vi "display queue.vi"(7 "Action":T1=enum."Enqueue", 8 "error in (no error)":errorcluster, 10 "time out":i32=100, 11 "Array in":sgl[](array[numeric])) -> (0 "error out":errorcluster, 1 "Array out":sgl[](array[numeric]), 2 "Empty?":bool, 3 "timed out?":bool)   [LabVIEW 2018]
uses:
  Controls/Queue Manager Actions.ctl
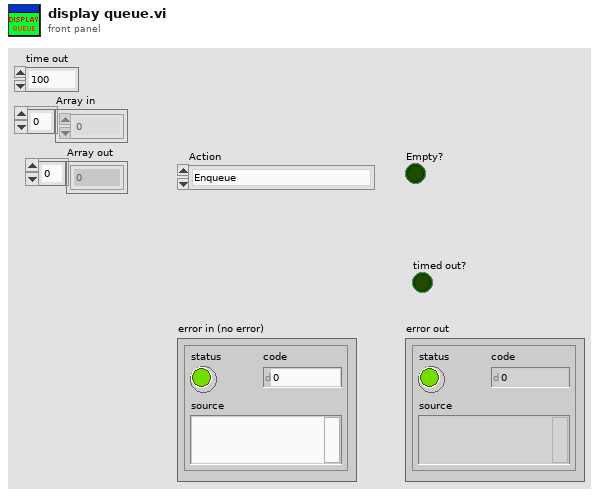
[diagram p1: front panel]
types:
  T1 = typedef "Queue Manager Actions.ctl" = enum16{"Init", "Enqueue", "Enqueue All", "Preview Queue", "Dequeue", "Get Status", "Flush Queue", "Flush All Queues", "Release All Queues", "Release Queue", "Enqueue at Opposite End"}
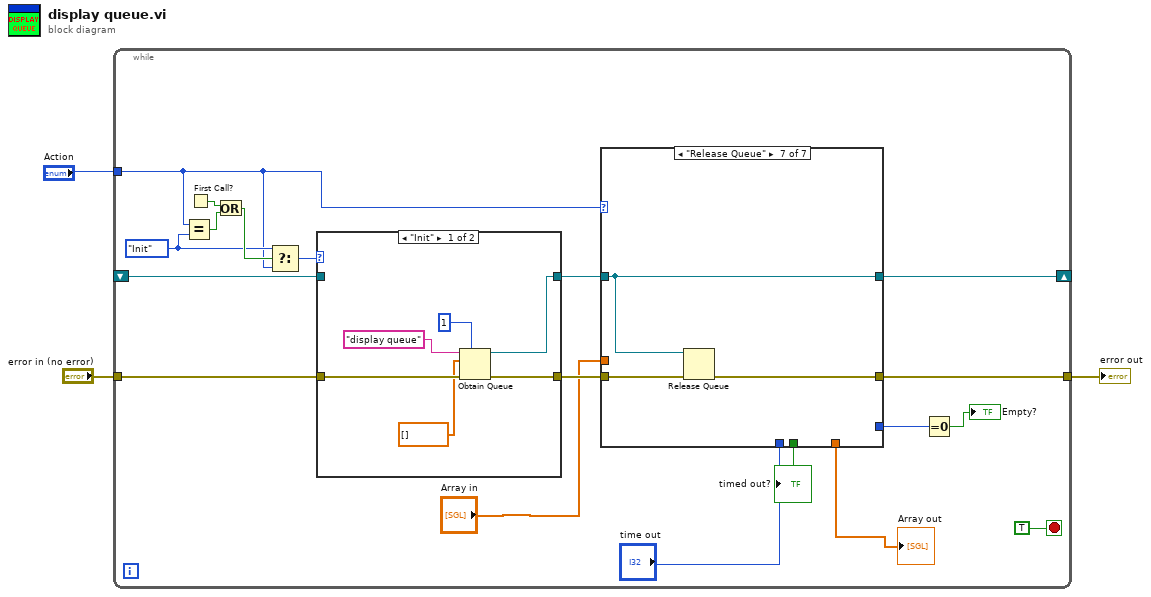
[diagram p0: block diagram]
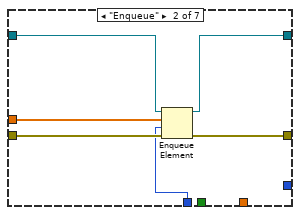
[diagram p3: hidden frame]
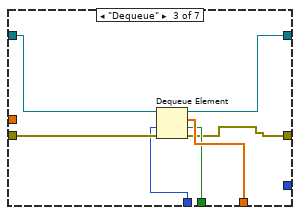
[diagram p4: hidden frame]
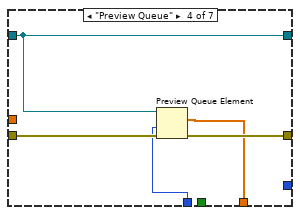
[diagram p5: hidden frame]
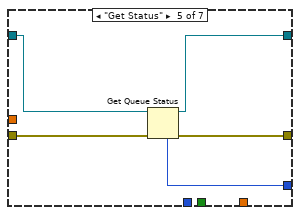
[diagram p6: hidden frame]
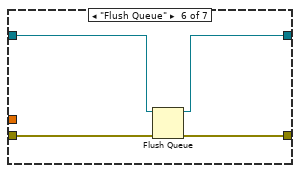
[diagram p7: hidden frame]
diagram:
  n1 = while {
    tunnel: "Action" -> [w10]
    tunnel: "error in (no error)" -> [w17]
    tunnel: [w16] -> w1
    shift-right: [w12] -> _
    shift-left: _ -> [w11]
    stop <- TRUE stop-if-true
    w19 = Queue_Manager_Actions."Init"
    n2 = Equal?(x=w10, y=w19) -> (x = y?=w21:bool)
    n3 = First Call?() -> (First Call?: T/F=w22:bool)
    n4 = Or(x=w22, y=w21) -> (x .or. y?=w20:bool)
    n5 = Select(t=w19, s=w20, f=w10) -> (s? t:f=w18:T1)
    n6 = case shown="\"Init\"" w18 {
      tunnel: [w60 w61] -> w14
      tunnel: w17 -> [w59 w62]
      tunnel: [w58 w62] -> w15
      tunnel: w11 -> [_ w61]
      frame "Init" {
        n7 = Obtain Queue(max queue size (-1, unlimited)=1, name (unnamed)="display queue" ("queue name"), element data type=sgl[] [], error in (no error)=w59) -> (queue out=w60:refnum<queue>, error out=w58:errorcluster)  [unwired: 1 in, 1 out]
      }
      frame "Enqueue", Default {
      }
    }
    n8 = case shown="\"Release Queue\"" w10 {
      tunnel: w14 -> [w23 w26 w35 w39 w45 w49 w52]
      tunnel: [w24 w29 w31 w41 w46 w50 w53] -> w16
      tunnel: w15 -> [w24 w30 w37 w42 w47 w51 w54]
      tunnel: [w23 w25 w32 w39 w44 w48 w52] -> w12
      tunnel: "time out" -> [_ w28 w36 w40 _ _ _]
      tunnel: "Array in" -> [_ w27 _ _ _ _ _]
      tunnel: [_ _ _ _ w43 _ _] -> w8
      tunnel: [_ _ w34 w38 _ _ _] -> w4
      tunnel: [_ _ w33 _ _ _ _] -> w7
      frame "Init", Default {
      }
      frame "Enqueue" {
        n9 = Enqueue Element(queue=w26, element=w27, timeout in ms (-1)=w28, error in (no error)=w30) -> (queue out=w25:refnum<queue>, error out=w29:errorcluster)  [unwired: 1 out]
      }
      frame "Dequeue" {
        n10 = Dequeue Element(queue=w35, timeout in ms (-1)=w36, error in (no error)=w37) -> (queue out=w32:refnum<queue>, element=w34:sgl[], timed out?=w33:bool, error out=w31:errorcluster)
      }
      frame "Preview Queue" {
        n11 = Preview Queue Element(queue=w39, timeout in ms (-1)=w40, error in (no error)=w42) -> (element=w38:sgl[], error out=w41:errorcluster)  [unwired: 2 out]
      }
      frame "Get Status" {
        n12 = Get Queue Status(queue=w45, error in (no error)=w47) -> (queue out=w44:refnum<queue>, error out=w46:errorcluster, # elements in queue=w43:i32)  [unwired: 1 in, 5 out]
      }
      frame "Flush Queue" {
        n13 = Flush Queue(queue=w49, error in (no error)=w51) -> (queue out=w48:refnum<queue>, error out=w50:errorcluster)  [unwired: 1 out]
      }
      frame "Release Queue" {
        n14 = Release Queue(queue=w52, error in (no error)=w54) -> (error out=w53:errorcluster)  [unwired: 1 in, 2 out]
      }
    }
    "timed out?" <- w7
    "Array out" <- w4
    n15 = Equal To 0?(x=w8) -> (x = 0?=→"Empty?":bool)
  }
  "error out" <- w1
